vi "SetRenderTarget.vi"(8 "No Error":errorcluster, 10 "texture [SDL_Texture *]":i64, 11 "renderer [SDL_Renderer *]":i64) -> (0 "error out":errorcluster)   [LabVIEW 2024, in "SDL3.lvlib" / "Render.lvlib"]
doc: "<B>Summary</B>\nSet a texture as the current rendering target.\n\n<B>Remarks</B>\nThe default render target is the window for which the renderer was created. To stop rendering to a texture and render to the window again, call this function with a NULL texture.\n\n<B>Thread Safety</B>\nYou may only call this function from the main thread."
uses:
  Render.lvlib
  Error/Error.lvlib
  Lib/SDL3-32.dll
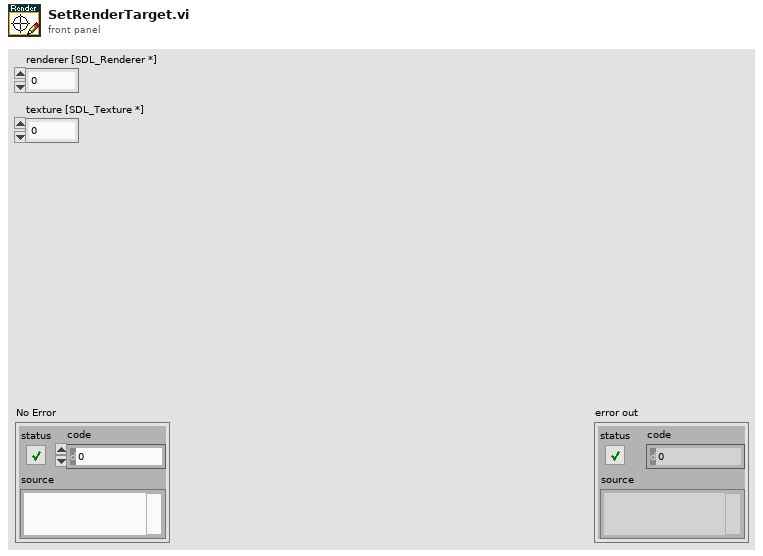
[diagram p1: front panel]
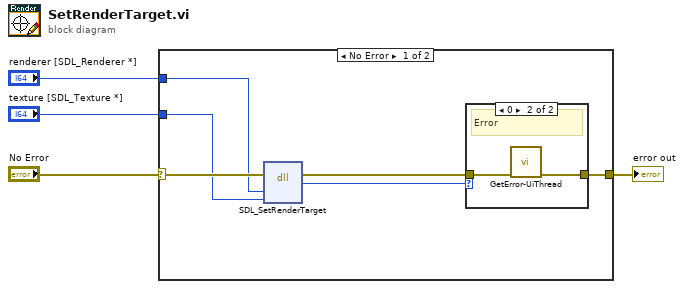
[diagram p0: block diagram]
diagram:
  n1 = case shown="No Error" "No Error" {
    selector: "No Error" -> [w10 w14]
    tunnel: [w8 w14] -> w3
    tunnel: "renderer [SDL_Renderer *]" -> [w6 _]
    tunnel: "texture [SDL_Texture *]" -> [w5 _]
    frame No Error {
      n2 = dll-call lib="C:/Users/Thomas/Documents/Projects/LV-SDL3/Lib/SDL3-*.*" fn="SDL_SetRenderTarget"(error in=w10, "renderer"=w6, "texture"=w5) -> (error out=w9:errorcluster, "return type"=w7:i32)  [unwired: 4 in, 1 out]
      n3 = case shown="0" w7 {
        tunnel: w9 -> [w11 w13]
        tunnel: [w11 w12] -> w8
        frame Default {
          # "Ok"
        }
        frame 0 {
          # "Error"
          n4 = call "GetError-UiThread.vi"("No Error"=w13) -> ("error out"=w12:errorcluster)  [unwired: 10 in]
        }
      }
    }
    frame Error {
    }
  }
  "error out" <- w3
